vi "ZPL Initialize.vi"(6 "Language Selector":i16(ring)=1 items=["GEN", "SCPI"], 7 "Address":i16=6, 8 "error in":errorcluster, 9 "ID Query (T)":bool=TRUE, 10 "Baud Rate":i32(ring)=3 items=["1200", "2400", "4800", "9600", "19200", "38400", "57600", "115200"], 11 "VISA":refnum<visa-resource-name>) -> (0 "error out":errorcluster, 3 "VISA  out":refnum<visa-resource-name>, 4 "ID responce":string, 5 "Address \"OK\"":string)   [LabVIEW 2016]
doc: "This VI passes the addressing information in the instrument decriptor to the Instr Open VI and returns the instrument ID. You can optionally reset the instrument by setting the front panel reset control. You must run this VI before using any of the instrument driver VIs for this instrument."
uses:
  <vilib>/Instr/_visa.llb/VISA Open Access Mode.ctl
panel:
  # "Initialize Instrument\nOpen VISA Port"
  # "Lambda ZPLUS \n  DC Power Supplies"
  # "Reset\nDon't Reset"
  # "Check\nDon't Check"
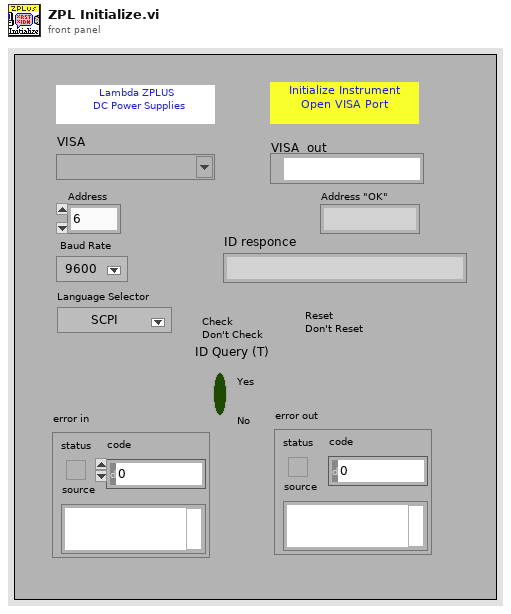
[diagram p1: front panel]
types:
  T1 = typedef "VISA Open Access Mode.ctl" = u32
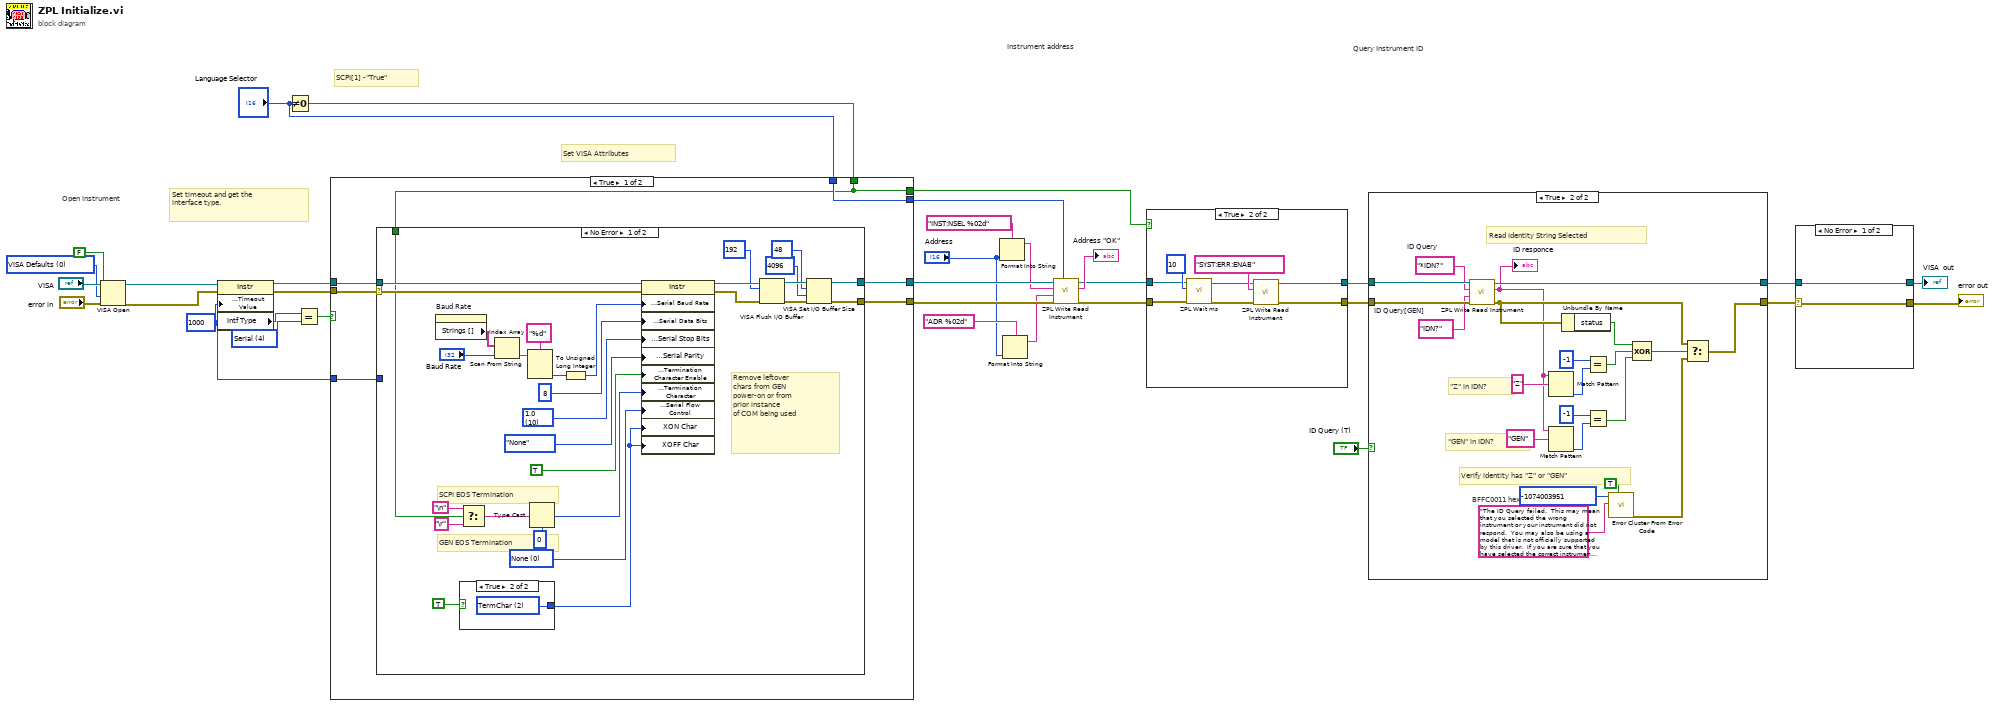
[diagram p0: block diagram]
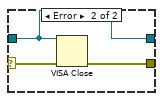
[diagram p3: hidden frame]
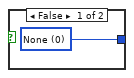
[diagram p5: hidden frame]
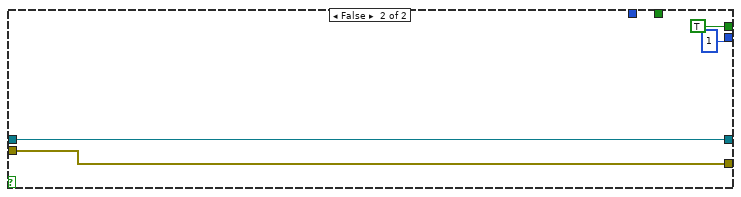
[diagram p7: hidden frame]
diagram:
  w23 = T1 0 items=["VISA Defaults"=0, "Exclusive Lock"=1, "Load Configured Settings"=4] ("Access Mode")
  w30 = u16 4 items=["GPIB"=1, "VXI"=2, "GPIB-VXI"=3, "Serial"=4, "PXI"=5, "TCPIP"=6, "USB"=7] ("Interface Information:Interface Type")
  w13 = u32 1000 ("Tmo Value")
  # "SCPI[1] -\"True\""
  # "Query Instrument ID"
  # "Set VISA Attributes"
  # "Instrument address"
  # "Set timeout and get the\ninterface type."
  # "Open instrument"
  n1 = VISA Open(duplicate session (F)=FALSE, access mode=w23, error in (no error)="error in", VISA resource name="VISA") -> (VISA resource name=w12:refnum<visa-resource-name>, error out=w11:errorcluster)  [unwired: 1 in]
  n2 = property class="Instr"(reference=w12, error in=w11, "General Settings:Timeout Value"=w13) -> (reference out=w31:refnum<visa-resource-name>, error out=w32:errorcluster, "Intf Type"=w29:u16)
  n3 = Not Equal To 0?(x="Language Selector") -> (x != 0?=w2:bool)
  n4 = Equal?(x=w29, y=w30) -> (x = y?=w28:bool)
  n5 = case shown="True" w28 {
    tunnel: w32 -> [w37 w77]
    tunnel: w31 -> [w40 w78]
    tunnel: [w39 w78] -> w27
    tunnel: [w38 w77] -> w26
    tunnel: w13 -> [w36 _]
    tunnel: [w34 TRUE] -> w1
    tunnel: w2 -> [w34 _]
    tunnel: "Language Selector" -> [w35 _]
    tunnel: [w35 i16 1 ("Language Selector")] -> w3
    frame True {
      n6 = case shown="No Error" w37 {
        selector: w37 -> [w61 w74]
        tunnel: w40 -> [w65 w73]
        tunnel: [w58 w73] -> w39
        tunnel: [w57 w74] -> w38
        tunnel: w34 -> [w49 _]
        tunnel: w36 -> [_ _]
        frame No Error {
          w68 = u16 10 items=["1.0"=10, "1.5"=15, "2.0"=20] ("stop bits (10: 1 bit)")
          w66 = u16 0 items=["None", "XON/XOFF", "RTS/CTS", "XON/XOFF & RTS/CTS", "DTR/DSR", "XON/XOFF & DTR/DSR"] ("flow control (0:none)")
          # "SCPI EOS Termination"
          # "GEN EOS Termination"
          # "Remove leftover\nchars from GEN\npower-on or from\nprior instance\nof COM being used"
          n7 = property on="Baud Rate" class="Ring (strict)"() -> ("Strings []"=w56:string[])  [unwired: 2 in, 2 out]
          n8 = case shown="True" TRUE {
            tunnel: [w71 w72] -> w42
            frame False {
              w71 = u16 0 items=["None", "LastBit", "TermChar"] ("Serial Settings:Serial End Mode for Reads")
            }
            frame True {
              w72 = u16 2 items=["None", "LastBit", "TermChar"] ("Serial Settings:Serial End Mode for Reads")
            }
          }
          n9 = Select(t="\n", s=w49, f="\r") -> (s? t:f=w52:string)
          n10 = Index Array(array=w56, index="Baud Rate") -> (element=w53:string)
          n11 = Scan From String(format string="%d", input string=w53) -> (output 1=w55:i32)  [unwired: 3 in, 3 out]
          n12 = Type Cast(type=u8 0, x=w52) -> (*(type *) &x=w62:u8)
          n13 = To Unsigned Long Integer(number=w55) -> (unsigned 32bit integer=w41:u32)
          n14 = property class="Instr"(reference=w65, error in=w61, "Serial Settings:Serial Baud Rate"=w41, "Serial Settings:Serial Data Bits"=u16 8 ("data bits (8)"), "Serial Settings:Serial Stop Bits"=w68, "Serial Settings:Serial Parity"=enum16{"None", "Odd", "Even", "Mark", "Space"}."None" ("parity (0:none)"), "Message Based Settings:Termination Character Enable"=TRUE ("Enable Termination\nChar (T)"), "Message Based Settings:Termination Character"=w62, "Serial Settings:Serial Flow Control"=w66, "XON Char"=w42, "XOFF Char"=w42) -> (reference out=w59:refnum<visa-resource-name>, error out=w60:errorcluster)
          n15 = VISA Flush I/O Buffer(VISA resource name=w59, mask (16)=u16 192, error in (no error)=w60) -> (VISA resource name out=w48:refnum<visa-resource-name>, error out=w47:errorcluster)
          n16 = VISA Set I/O Buffer Size(VISA resource name=w48, mask (16)=u16 48, size (4096)=u32 4096 ("size (0)"), error in (no error)=w47) -> (VISA resource name out=w58:refnum<visa-resource-name>, error out=w57:errorcluster)
        }
        frame Error {
        }
      }
    }
    frame False {
    }
  }
  n17 = Format Into String(format string="INST:NSEL %02d", "Address") -> (resulting string=w5:string)  [unwired: 2 in, 1 out]
  n18 = Format Into String(format string="ADR %02d", "Address") -> (resulting string=w6:string)  [unwired: 2 in, 1 out]
  n19 = call "ZPL Write Read Instrument.vi"("Language"=w3, "error in"=w26, "Write Command/Query GEN"=w6, "Write Command/Query SCPI"=w5, "VISA"=w27) -> ("error out"=w16:errorcluster, "Response"=→"Address \"OK\"":string, "VISA  out"=w17:refnum<visa-resource-name>)  [unwired: 4 in]
  n20 = case shown="True" w1 {
    tunnel: w17 -> [w80 w85]
    tunnel: w16 -> [w79 w86]
    tunnel: [w80 w82] -> w15
    tunnel: [w79 w81] -> w14
    frame False {
    }
    frame True {
      n21 = call "ZPL Wait ms.vi"("error"=w86, "Delay (1 mS)"=u32 10, "VISA"=w85) -> ("error out"=w83:errorcluster, "VISA out"=w84:refnum<visa-resource-name>)  [unwired: 7 in]
      n22 = call "ZPL Write Read Instrument.vi"("error in"=w83, "Write Command/Query SCPI"="SYST:ERR:ENAB" ("Write Command/Query"), "VISA"=w84) -> ("error out"=w81:errorcluster, "VISA  out"=w82:refnum<visa-resource-name>)  [unwired: 6 in, 1 out]
    }
  }
  n23 = case shown="True" "ID Query (T)" {
    tunnel: w15 -> [w90 w112]
    tunnel: w14 -> [w89 w111]
    tunnel: [w90 w110] -> w24
    tunnel: [w89 w95] -> w21
    frame False {
    }
    frame True {
      w92 = "*IDN?"  # ID Query
      w91 = "IDN?"  # ID Query[GEN]
      # "BFFC0011 hex"
      # "\"GEN\" in IDN?"
      # "\"Z\" in IDN?"
      # "Verify identity has \"Z\" or \"GEN\""
      # "Read Identity String Selected"
      n24 = call "ZPL Write Read Instrument.vi"("error in"=w111, "Write Command/Query GEN"=w91, "Write Command/Query SCPI"=w92, "VISA"=w112) -> ("error out"=w96:errorcluster, "Response"=w94:string, "VISA  out"=w110:refnum<visa-resource-name>)  [unwired: 5 in]
      "ID responce" <- w94
      n25 = Match Pattern(string=w94, regular expression="Z") -> (offset past match=w107:i32)  [unwired: 1 in, 3 out]
      n26 = Match Pattern(string=w94, regular expression="GEN") -> (offset past match=w106:i32)  [unwired: 1 in, 3 out]
      n27 = Unbundle By Name(w96) -> ("status"=w103:bool)
      n28 = Equal?(x=-1, y=w107) -> (x = y?=w102:bool)
      n29 = Equal?(x=-1, y=w106) -> (x = y?=w101:bool)
      n30 = call <vilib>:"Error Cluster From Error Code.vi"("show call chain? (False)"=TRUE, "error message (\"\")"="The ID Query failed.  This may mean that you selected the wrong instrument or your instrument did not respond.  You may also be using a model that is not officially supported by this driver.  If you are sure that you have selected the correct instrument and it is responding, try disabling the ID Query." ("Source (VI Name)"), "error code (0)"=-1074003951 ("Code")) -> ("error out"=w97:errorcluster)  [unwired: 6 in]
      n31 = Compound Arithmetic op=XOR(w103, w102, w101) -> (w93:bool)
      n32 = Select(t=w96, s=w93, f=w97) -> (s? t:f=w95:errorcluster)
    }
  }
  n33 = case shown="No Error" w21 {
    selector: w21 -> [w114 w117]
    tunnel: w24 -> [w113 w115]
    tunnel: [w114 w116] -> w20
    tunnel: [w113 w115] -> w18
    frame No Error {
    }
    frame Error {
      n34 = VISA Close(VISA resource name=w115, error in (no error)=w117) -> (error out=w116:errorcluster)
    }
  }
  "VISA  out" <- w18
  "error out" <- w20
